vi "Add Virtual Instruments.vi"(8 "error in":errorcluster, 10 "<JSON> CFG":string, 11 "MSS in":refnum<class "MSS.lvclass">) -> (0 "error out":errorcluster, 2 "Target Virt Instrs":T1(array[cluster]), 3 "MSS out":refnum<class "MSS.lvclass">)   [LabVIEW 2023, in "HAL.lvlib" / "MSS.lvclass"]
uses:
  MSS.lvclass
  4d7fb90e-0f91-4117-ba7a-7e09055b6ec3.vi
  4d7fb90e-0f91-4117-ba7a-7e09055b6ec3.vi/a4169a97-72fc-4003-a778-603cf20cafa0.vi
  <vilib>/JDP Science/JSONtext/Find Item.vi
  <vilib>/JDP Science/JSONtext/Next JSON Value.vi
  <vilib>/JDP Science/JSONtext/String Subset.vi
  <vilib>/JDP Science/JSONtext/Parsing/Advance past next JSON Value (inlined COPY).vi
  <vilib>/JDP Science/JSONtext/Parsing/Advance past whitespace.vi
  <vilib>/JDP Science/JSONtext/Parsing/Advance past String.vi
  <vilib>/JDP Science/JSONtext/Parsing/Advance past Number.vi
  <vilib>/JDP Science/JSONtext/Parsing/Advance past Line Ending.vi
  <vilib>/JDP Science/JSONtext/Parsing/Parse Full Path or Item Name.vi
  <vilib>/JDP Science/JSONtext/Parsing/Advance past Array.vi
  <vilib>/JDP Science/JSONtext/Parsing/Advance past Object.vi
  <vilib>/JDP Science/JSONtext/support/Error Cluster From Code.vi
  <vilib>/JDP Science/JSONtext/Offset/Find Item Locations by Path.vi
  <vilib>/JDP Science/JSONtext/JSON text to Variant.vi
  <vilib>/Utility/error.llb/Error Cluster From Error Code.vi
  <vilib>/JDP Science/JSONtext/LVClass Serializer/JSONtext LVClass Serializer.lvclass
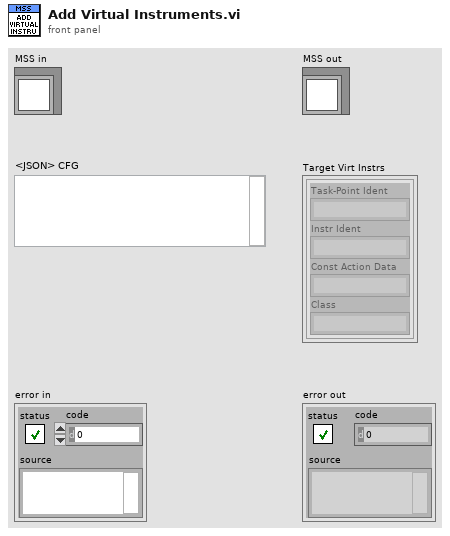
[diagram p1: front panel]
types:
  T1 = cluster{"Task-Point Ident":string, "Instr Ident":string, "Const Action Data":string, "Class":string}[]
  T2 = cluster{"Point Ident":string, "Instr Ident":string, "<JSON>Perform Action":string, "<JSON>Scaling":string}[]
  T3 = cluster{"Point Ident":string, "Instr Ident":string, "<JSON> Perform Action CFG":string, "<JSON> Scaling CFG":string}[]
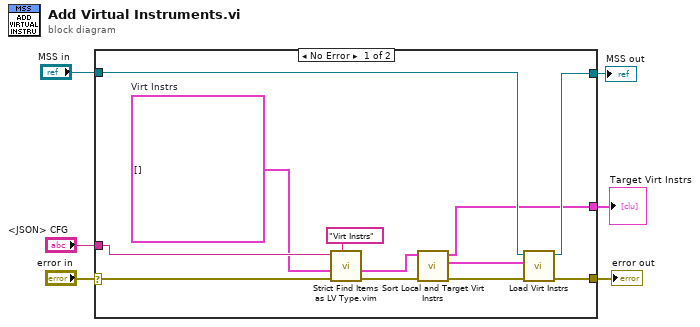
[diagram p0: block diagram]
diagram:
  n1 = case shown="No Error" "error in" {
    selector: "error in" -> [w14 w20]
    tunnel: [w18 w19] -> w6
    tunnel: [w17 w20] -> w5
    tunnel: "MSS in" -> [w16 w19]
    tunnel: "<JSON> CFG" -> [w15 _]
    tunnel: [w7 _] -> w1
    frame No Error {
      w13 = T2 []  # Virt Instrs
      n2 = call "Strict Find Items as LV Type.vim"("$Path or Item Name"="Virt Instrs", "error in"=w14, "Data Type and Default Value"=w13, "<JSON>"=w15) -> ("error out"=w10:errorcluster, "Data out"=w11:T2)  [unwired: 5 in, 1 out]
      n3 = call "Sort Local and Target Virt Instrs.vi"("error in"=w10, "Virt Instr CFGs"=w11) -> ("error out"=w9:errorcluster, "Local Virt Instrs"=w8:T3, "Target Virt Instrs"=w7:T2)  [unwired: 7 in]
      n4 = call "Load Virt Instrs.vi"("error in"=w9, "Local Virt Instrs"=w8, "MSS in"=w16) -> ("error out"=w17:errorcluster, "MSS out"=w18:refnum<class "MSS.lvclass">)  [unwired: 7 in]
    }
    frame Error {
    }
  }
  "error out" <- w5
  "MSS out" <- w6
  "Target Virt Instrs" <- w1
